vi "Shutdown cameras.vi"   [LabVIEW 2012]
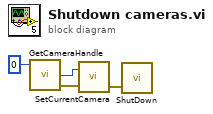
[diagram p0: block diagram]
diagram:
  n1 = call <userlib>:"GetCameraHandle.vi"("cameraIndex"=0) -> ("error out"=w3:errorcluster, "cameraHandle"=w1:i32)  [unwired: 2 in, 1 out]
  n2 = call <userlib>:"SetCurrentCamera.vi"("error in (no error)"=w3, "cameraHandle"=w1) -> ("error out"=w4:errorcluster)  [unwired: 1 out]
  n3 = call <userlib>:"ShutDown.vi"("error in (no error)"=w4) -> ()  [unwired: 1 in, 2 out]
